vi "Verificar_Posicion_En_Pistas.vi"(2 "Pistas":T1(array[cluster]), 3 "Posicion":string) -> (0 "Indice_Pista":dbl, 1 "Es_Una_Pista":bool)   [LabVIEW 2019]
doc: "Verifica si la 'Posicion' de tipo String 'x,y' se encuentra en la lista de pistas, si la encuentra retorna True y el indide de la imagen de la pista."
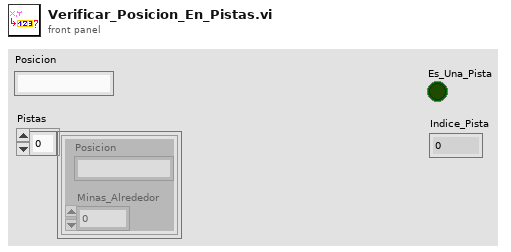
[diagram p1: front panel]
types:
  T1 = cluster{"Posicion":string, "Minas_Alrededor":dbl}[]
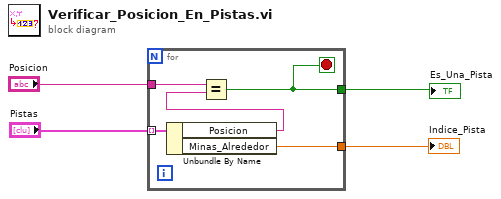
[diagram p0: block diagram]
diagram:
  n1 = for {
    tunnel: "Pistas" -> [w9] mode=indexing
    tunnel: "Posicion" -> [w7]
    tunnel: [w6] -> w4
    tunnel: [w5] -> w1
    stop <- w6 stop-if-true
    n2 = Unbundle By Name(w9) -> ("Posicion"=w8:string, "Minas_Alrededor"=w5:dbl)
    n3 = Equal?(x=w7, y=w8) -> (x = y?=w6:bool)
  }
  "Es_Una_Pista" <- w4
  "Indice_Pista" <- w1
